vi "GetDriveValuesFromAngle.vi"(2 "Rotate_To":dbl, 3 "Distance_To_Go":dbl) -> (0 "Right":dbl, 1 "Left":dbl)   [LabVIEW 2015]
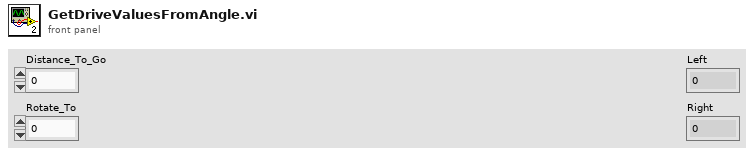
[diagram p1: front panel]
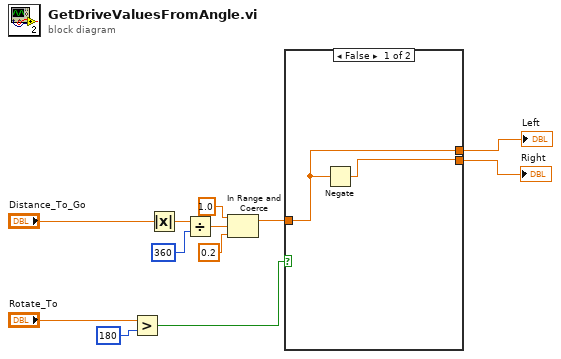
[diagram p0: block diagram]
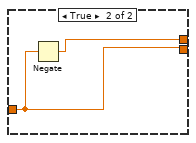
[diagram p2: hidden frame]
diagram:
  n1 = Greater?(x="Rotate_To", y=180) -> (0:w6:bool)
  n2 = Absolute Value(x="Distance_To_Go") -> (abs(x)=w12:dbl)
  n3 = Divide(x=w12, y=360) -> (x/y=w10:dbl)
  n4 = In Range and Coerce(upper limit=1.0, x=w10, lower limit=0.2) -> (coerced(x)=w5:dbl)  [unwired: 1 out]
  n5 = case shown="False" w6 {
    tunnel: w5 -> [w14 w15]
    tunnel: [w14 w16] -> w4
    tunnel: [w13 w15] -> w3
    frame False {
      n6 = Negate(x=w14) -> (-x=w13:dbl)
    }
    frame True {
      n7 = Negate(x=w15) -> (-x=w16:dbl)
    }
  }
  "Left" <- w4
  "Right" <- w3
